vi "RS_RF_move.vi"(1 "Points":cluster{string, "data":u64, "data":dbl}, 2 "Instr. Info":T1) -> ()   [LabVIEW 2013]
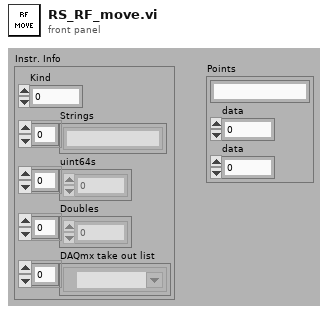
[diagram p1: front panel]
types:
  T1 = cluster{"Kind":u16, "Strings":string[], "uint64s":u64[], "Doubles":dbl[], "DAQmx take out list":refnum<k21>[]}
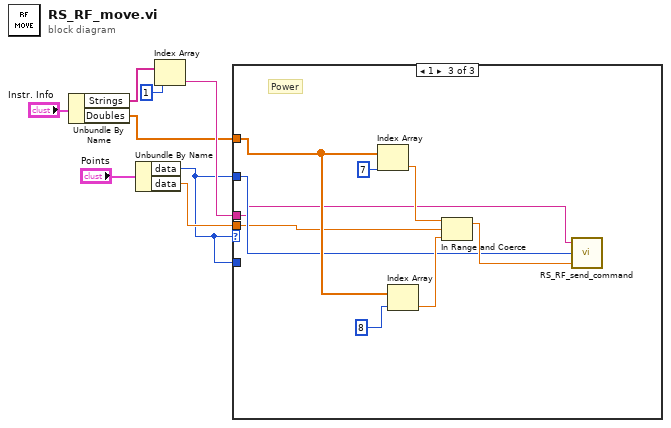
[diagram p0: block diagram]
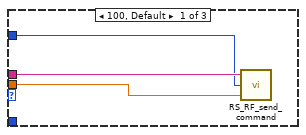
[diagram p2: hidden frame]
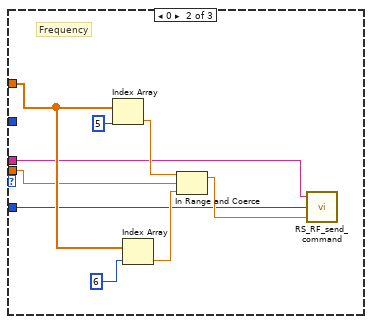
[diagram p3: hidden frame]
diagram:
  n1 = Unbundle By Name("Instr. Info") -> ("Strings"=w6:string[], "Doubles"=w2:dbl[])
  n2 = Unbundle By Name("Points") -> ("data"=w1:u64, "data"=w3:dbl)
  n3 = Index Array(array=w6, index=1) -> (element=w4:string)
  n4 = case shown="1" w1 {
    tunnel: w4 -> [w11 w13 w21]
    tunnel: w3 -> [w10 w17 w22]
    tunnel: w1 -> [w9 _ w23]
    tunnel: w2 -> [_ w20 w24]
    tunnel: w1 -> [_ w12 _]
    frame 100, Default {
      n5 = call "RS_RF_send_command.vi"("Value"=w10, "Parameter"=w9, "GPIB address"=w11) -> ()  [unwired: 1 in]
    }
    frame 0 {
      # "Frequency"
      n6 = Index Array(array=w20, index=5) -> (element=w16:dbl)
      n7 = Index Array(array=w20, index=6) -> (element=w15:dbl)
      n8 = In Range and Coerce(upper limit=w16, x=w17, lower limit=w15) -> (coerced(x)=w14:dbl)  [unwired: 1 out]
      n9 = call "RS_RF_send_command.vi"("Value"=w14, "Parameter"=w12, "GPIB address"=w13) -> ()  [unwired: 1 in]
    }
    frame 1 {
      # "Power"
      n10 = Index Array(array=w24, index=7) -> (element=w27:dbl)
      n11 = Index Array(array=w24, index=8) -> (element=w26:dbl)
      n12 = In Range and Coerce(upper limit=w27, x=w22, lower limit=w26) -> (coerced(x)=w25:dbl)  [unwired: 1 out]
      n13 = call "RS_RF_send_command.vi"("Value"=w25, "Parameter"=w23, "GPIB address"=w21) -> ()  [unwired: 1 in]
    }
  }
